vi "GetLinks.vi"() -> ()   [LabVIEW 2012]
uses:
  <userlib>/ROSforLV/ROS/Code/SubVIs/_ROSDirection.ctl
  <userlib>/ROSforLV/ROS/Code/_ROSDefinition.vi
panel:
  in  "Set New Pose":bool
  in  "Refresh Links?":bool
  in  "New Twist":T1
  in  "New Pose":T2
  out "Twists":T3(array[cluster])
  out "Poses":T4(array[cluster]) {"Point"."y" format="%#_3f"}
  in  "Link To Move":string(combo)
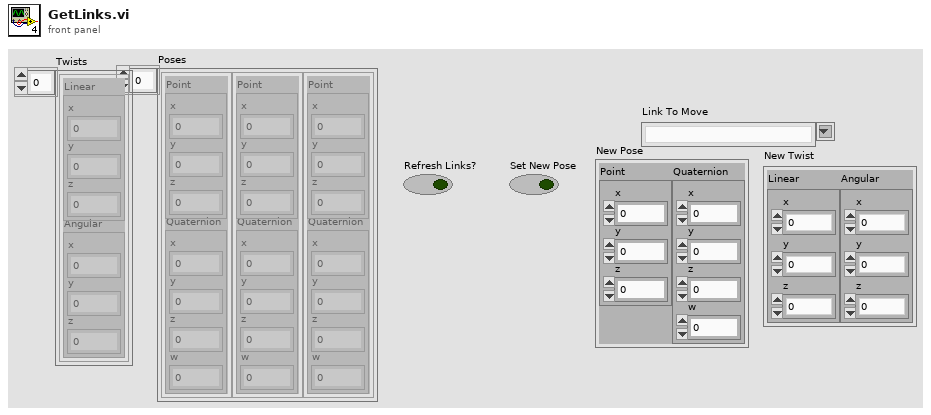
[diagram p1: front panel]
types:
  T1 = cluster{"Linear":cluster{"x":dbl, "y":dbl, "z":dbl}, "Angular":cluster{"x":dbl, "y":dbl, "z":dbl}}
  T2 = cluster{"Point":cluster{"x":dbl, "y":dbl, "z":dbl}, "Quaternion":cluster{"x":dbl, "y":dbl, "z":dbl, "w":dbl}}
  T3 = cluster{"Linear":cluster{"x":dbl, "y":dbl, "z":dbl}, "Angular":cluster{"x":dbl, "y":dbl, "z":dbl}}[]
  T4 = cluster{"Point":cluster{"x":dbl, "y":dbl, "z":dbl}, "Quaternion":cluster{"x":dbl, "y":dbl, "z":dbl, "w":dbl}}[]
  T5 = typedef "_ROSDirection.ctl" = enum16{"Node", "Publisher", "Subscriber", "Service Client"}
  T6 = cluster{"Topic":string, "Type":string, "Action":T5, "Update (ms)":u16, "write queue":u16}
  T7 = typedef "_ROSControl.ctl" = cluster{"topic port":u16, "Node":string, "topic":string, "type":string, "node port":u32, "error ":errorcluster, "Direction":T5, "APIs":string[], "Update (ms)":u16, "write queue":u16}
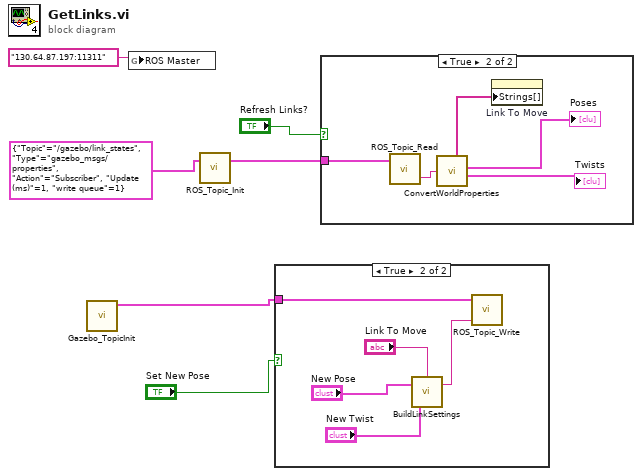
[diagram p0: block diagram]
diagram:
  n1 = call <userlib>:"Gazebo_TopicInit.vi"() -> ("ROS out"=w4:T7)  [unwired: 11 in]
  n2 = global write "_ROSDefinition.vi" "ROS Master"("130.64.87.197:11311" ("ROS Master")) -> ()
  n3 = call <userlib>:"ROS_Topic_Init.vi"("Definitions"=T6 {"Topic"="/gazebo/link_states", "Type"="gazebo_msgs/properties", "Action"=enum."Subscriber", "Update (ms)"=1, "write queue"=1} ("element")) -> ("ROS out"=w5:T7)  [unwired: 2 in]
  n4 = case shown="True" "Set New Pose" {
    tunnel: w4 -> [_ w7]
    frame False {
    }
    frame True {
      n5 = call <userlib>:"BuildLinkSettings.vi"("Twist"="New Twist", "Pose"="New Pose", "link to move"="Link To Move") -> ("msg out"=w8:string)  [unwired: 1 in]
      n6 = call <userlib>:"ROS_Topic_Write.vi"("Msg in"=w8, "ROS in"=w7) -> ()  [unwired: 2 in, 1 out]
    }
  }
  n7 = case shown="True" "Refresh Links?" {
    tunnel: w5 -> [_ w16]
    frame False {
    }
    frame True {
      n8 = call <userlib>:"ROS_Topic_Read.vi"("ROS in"=w16) -> ("Reply"=w15:string)  [unwired: 1 in, 1 out]
      n9 = call <userlib>:"ConvertWorldProperties.vi"("Reply"=w15) -> ("Poses"=→"Poses":T4, "Twists"=→"Twists":T3, "names"=w12:string[])  [unwired: 1 in, 1 out]
      n10 = property on="Link To Move" class="CmbBox"("Strings[]"=w12) -> ()  [unwired: 2 in, 2 out]
    }
  }
